vi "浮点数约等.vi"(1 "浮点数2":dbl format="%.2f", 2 "浮点数1":dbl format="%.2f") -> (0 "约等 ?":bool)   [LabVIEW 2012]
doc: "功能：\n\n判断两个浮点数是否大致相等，直接用=函数判断两个浮点数是否相等，因为存在精度问题，往往会导致错误结果。\n\n基本算法：\n\n当两个输入浮点数等于0时，判断两个数是否小于最小机器数。当两个浮点数不等于0时，利用两个数的绝对值做除法，结果在1上下某个范围时，认为两个浮点数相等。"
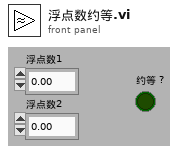
[diagram p1: front panel]
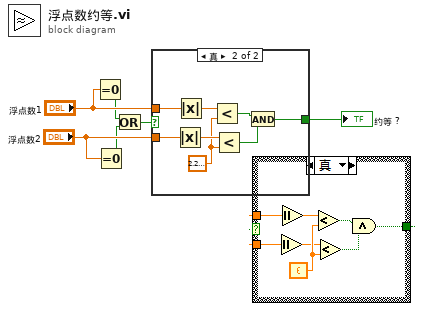
[diagram p0: block diagram]
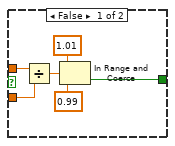
[diagram p2: hidden frame]
diagram:
  n1 = Equal To 0?(x="浮点数1") -> (x = 0?=w2:bool)
  n2 = Equal To 0?(x="浮点数2") -> (x = 0?=w3:bool)
  n3 = Or(x=w2, y=w3) -> (x .or. y?=w1:bool)
  n4 = case shown="真" w1 {
    tunnel: [w9 w14] -> w6
    tunnel: "浮点数2" -> [w8 w19]
    tunnel: "浮点数1" -> [w7 w20]
    frame False {
      n5 = Divide(x=w7, y=w8) -> (x/y=w12:dbl)
      n6 = In Range and Coerce(upper limit=1.01, x=w12, lower limit=0.99) -> (In Range?=w9:bool)  [unwired: 1 out]
    }
    frame True {
      w13 = 2.220446049250313e-16
      n7 = Absolute Value(x=w19) -> (abs(x)=w17:dbl)
      n8 = Absolute Value(x=w20) -> (abs(x)=w18:dbl)
      n9 = Less?(x=w18, y=w13) -> (x < y?=w16:bool)
      n10 = Less?(x=w17, y=w13) -> (x < y?=w15:bool)
      n11 = And(x=w16, y=w15) -> (x .and. y?=w14:bool)
    }
  }
  "约等 ?" <- w6
